vi "test_toml.vi"() -> (0 "error out":errorcluster, 2 "tests":bool[](array[boolean]), 3 "passed":bool)   [LabVIEW 2017]
uses:
  58c06032-3e23-4c53-85e7-224e0a2187e2.vi
  toml/value_boolean.vi
  toml/rpacini_toml.lvlib
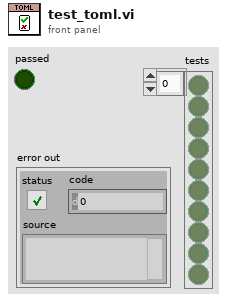
[diagram p1: front panel]
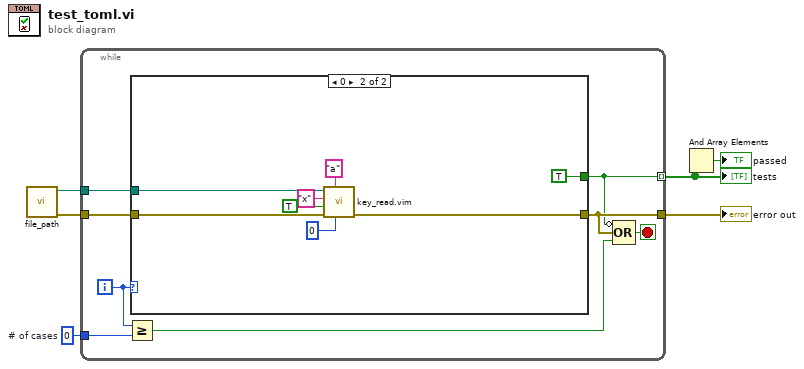
[diagram p0: block diagram]
diagram:
  w4 = 0  # # of cases
  n1 = call "file_path.vi"() -> ("error out"=w1:errorcluster, "app toml path"=w6:path)  [unwired: 8 in, 2 out]
  n2 = while {
    tunnel: w6 -> [w14]
    tunnel: w1 -> [w13]
    tunnel: [w12] -> w5
    tunnel: [w10] -> w3 mode=indexing
    tunnel: w4 -> [w8]
    i -> [w9]
    stop <- w11 stop-if-true
    n3 = Greater Or Equal?(x=w9, y=w8) -> (x >= y?=w7:bool)
    n4 = case shown="0" w9 {
      tunnel: w14 -> [_ w23]
      tunnel: w13 -> [w15 w22]
      tunnel: [w15 w21] -> w12
      tunnel: [_ TRUE] -> w10
      frame Default {
      }
      frame 0 {
        n5 = call "key_read.vim"("modifiers"=u16 0 ("modifiers (default)"), "section [str,1d,pth]"="a", "error in (no error)"=w22, "default [any]"=TRUE, "key [str,1d,pth]"="x", "path in"=w23) -> ("error out"=w21:errorcluster)  [unwired: 2 in, 3 out]
      }
    }
    n6 = Compound Arithmetic op=OR(invert w10, w12, w7) -> (w11:bool)
  }
  "error out" <- w5
  "tests" <- w3
  n7 = And Array Elements(Boolean array=w3) -> (logical AND=→"passed":bool)
